vi "Show Hide Items.vi"(7 "VI Ref":refnum<vi>, 8 "Error":errorcluster, 11 "(FP)":refnum<class "DecFrame_FP.lvclass">) -> (0 "Error Out":errorcluster, 3 "(FP) Out":refnum<class "DecFrame_FP.lvclass">, 5 "VI Ref Out":refnum<vi>)   [LabVIEW 2016, in "DecFrame_FP.lvclass"]
uses:
  DecFrame_FP.lvclass
  DecFrame_FP.lvclass/DecFrame_FP.ctl
  (FPEN)/(FPEN).lvclass
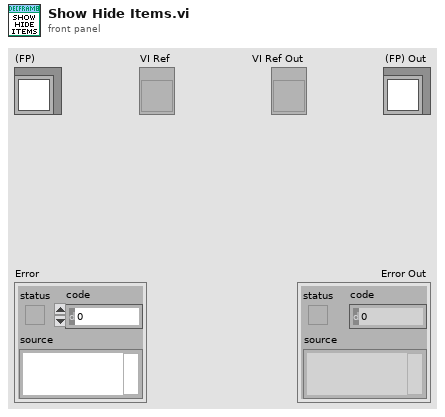
[diagram p1: front panel]
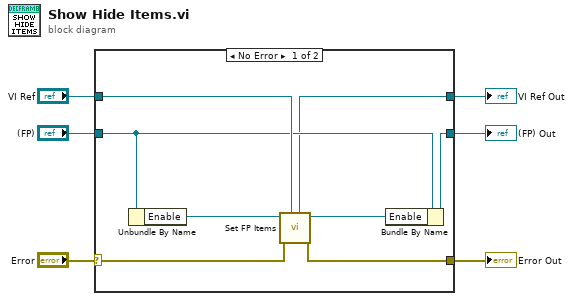
[diagram p0: block diagram]
diagram:
  n1 = case shown="No Error" "Error" {
    selector: "Error" -> [w13 w17]
    tunnel: [w7 w17] -> w5
    tunnel: [w11 w16] -> w3
    tunnel: "(FP)" -> [w12 w16]
    tunnel: "VI Ref" -> [w14 w15]
    tunnel: [w9 w15] -> w1
    frame No Error {
      n2 = Unbundle By Name(w12) -> ("Enable"=w10:refnum<class "(FPEN).lvclass">)
      n3 = call-dynamic "Set FP Items.vi"("VI Ref"=w14, "Error"=w13, "(FPEN)"=w10) -> ("Error Out"=w7:errorcluster, "(FPEN) Out"=w8:refnum<class "(FPEN).lvclass">, "VI Ref Out"=w9:refnum<vi>)  [unwired: 6 in]
      n4 = Bundle By Name(cluster=w12, "Enable"=w8) -> (w11:refnum<class "DecFrame_FP.lvclass">)
    }
    frame Error {
    }
  }
  "Error Out" <- w5
  "(FP) Out" <- w3
  "VI Ref Out" <- w1
